vi "conditioning monitor.vi"() -> ()   [LabVIEW 2016, in "Top Level.lvlib"]
doc: "takes the teminal voltage as well as the vacuum values for both the entrance and exit of accelerator. Display\nboth in long terminal graph form. Every 24 hours, the graph is cleared."
uses:
  Top Level.lvlib
  Controls/Vertical Rod states.ctl
panel:
  out "Current Time":string
  in  "reset":bool
  out "error out 2":errorcluster
  out "Start Time":string
  out "error out":errorcluster
  out "Terminal Voltage":cluster{"X":dbl[], "Y":dbl[]}[](graph)
  out "Tank Vacuum Pressures":cluster{"X":dbl[], "Y":dbl[]}[](graph)
  in  "Cluster":cluster{"X":dbl[], "Y":dbl[]}
  in  "stop":bool
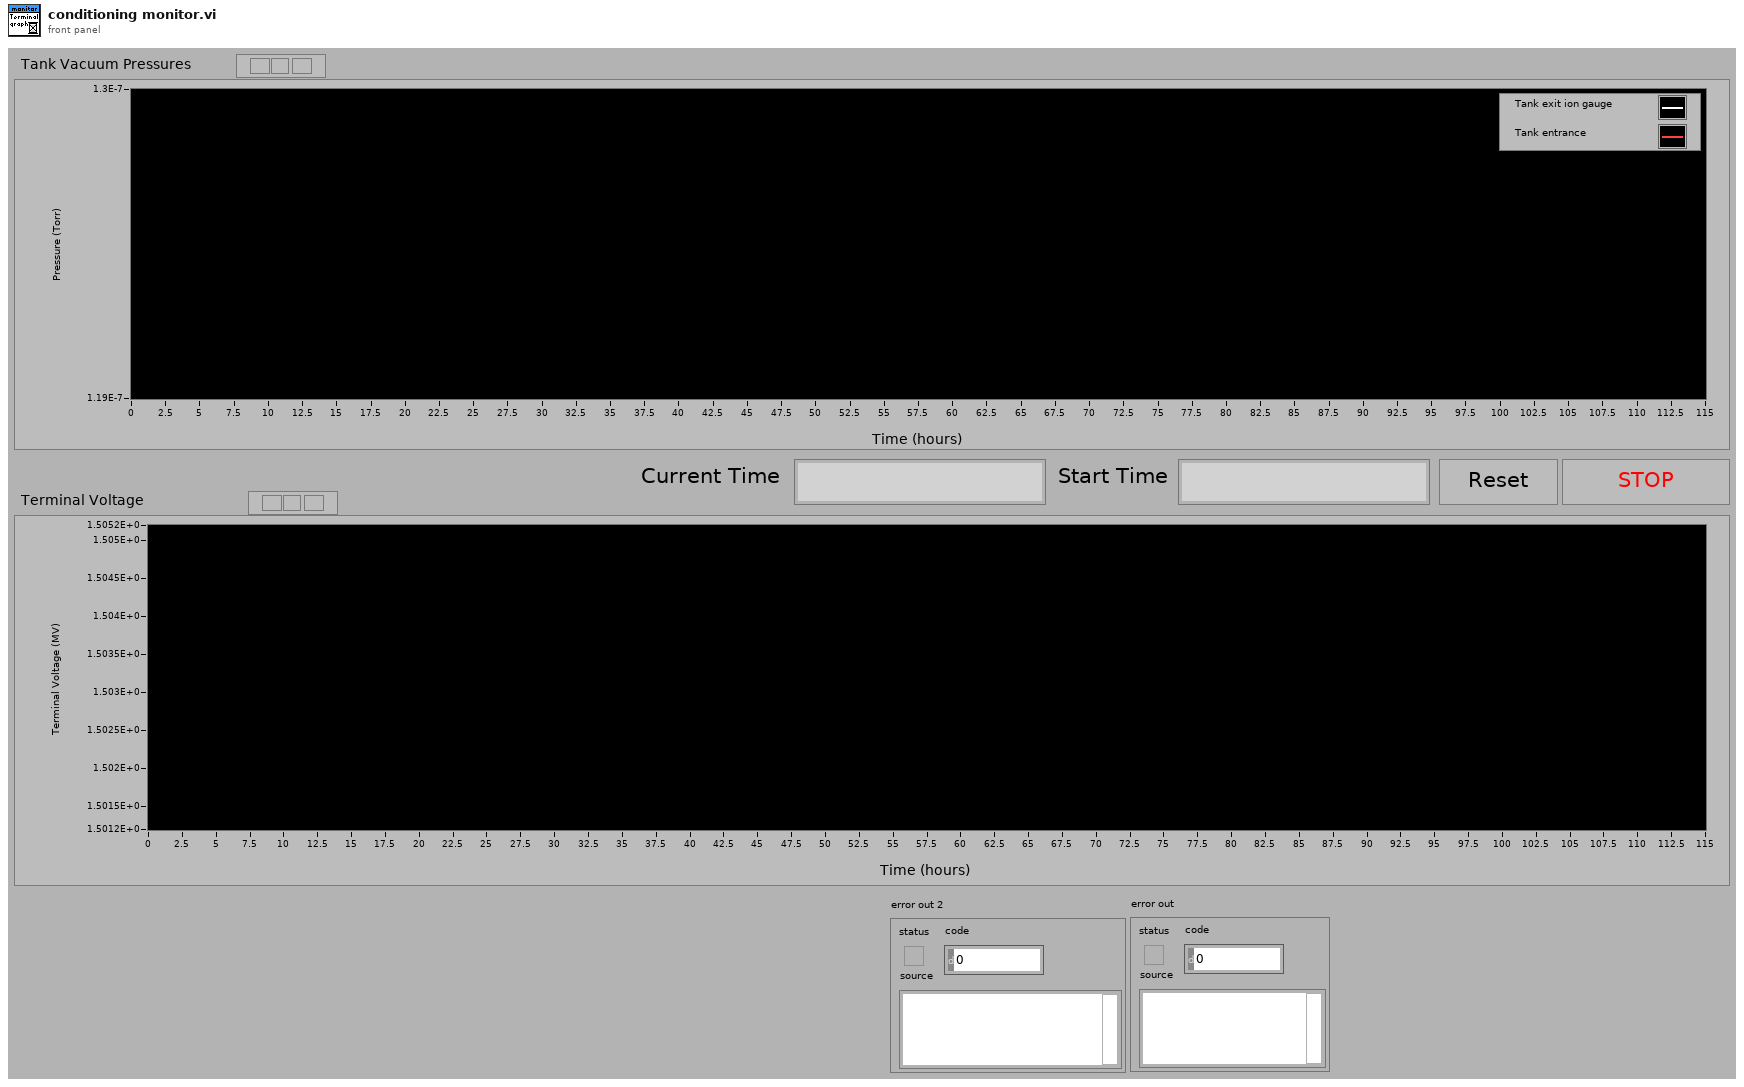
[diagram p1: front panel]
types:
  T1 = typedef "Vertical Rod states.ctl" = enum16{"status unclear", "rod down", "rod up"}
  T2 = cluster{"Ion gauge 1":string, "Convectron  Gauge 1 ":string, "Ion Gauge 2":string, "Convectrom Gauge 2":string}
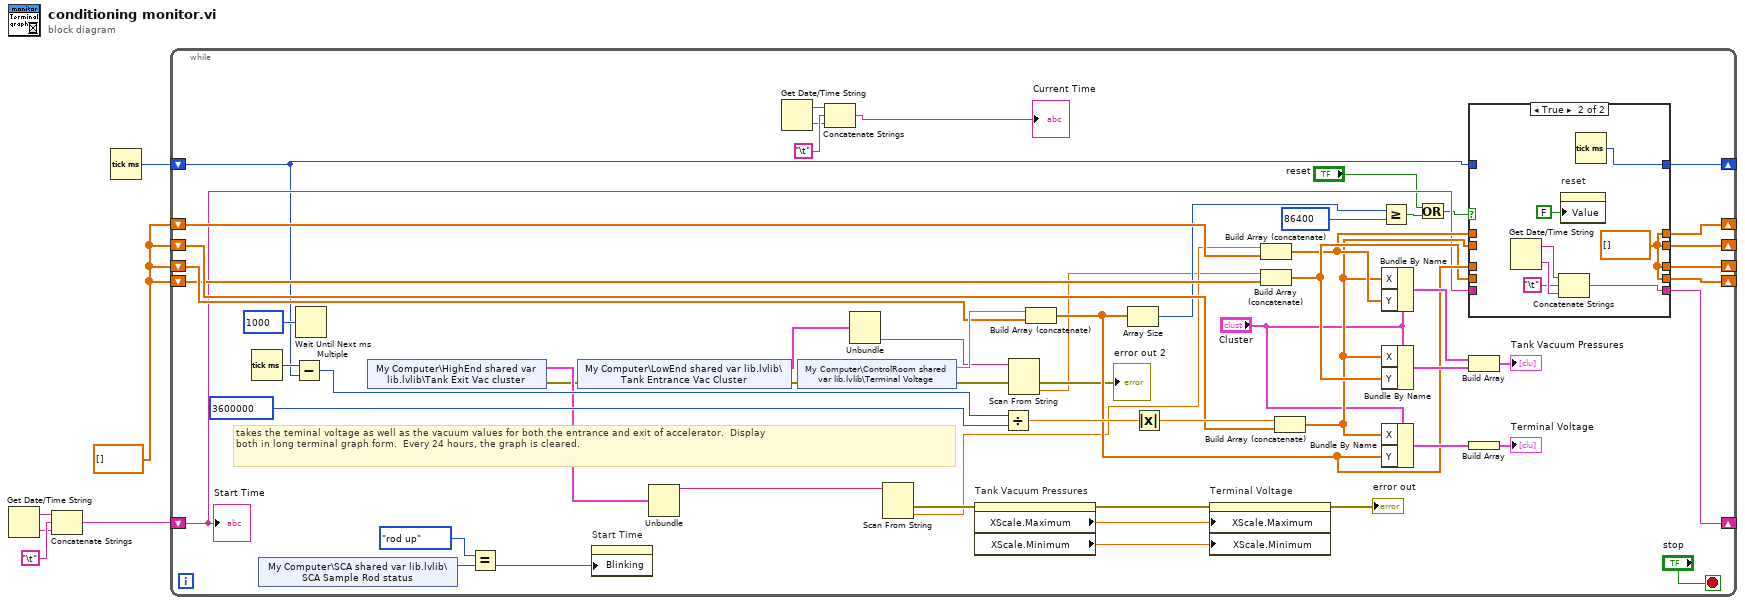
[diagram p0: block diagram]
diagram:
  w5 = dbl[] []
  n1 = Get Date/Time String() -> (date string=w4:string, time string=w2:string)  [unwired: 3 in]
  n2 = Concatenate Strings(w4, "\t", w2) -> (w1:string)
  n3 = Tick Count (ms)() -> (millisecond timer value=w6:u32)
  n4 = while {
    shift-right: [w27] -> _
    shift-left: w5 -> [w58]
    shift-right: [w25] -> _
    shift-left: w5 -> [w55]
    shift-right: [w31] -> _
    shift-left: w5 -> [w47]
    shift-right: [w29] -> _
    shift-left: w5 -> [w42]
    shift-right: [w24] -> _
    shift-left: w1 -> [w23]
    shift-right: [w13] -> _
    shift-left: w6 -> [w14]
    stop <- "stop" stop-if-true
    # "takes the teminal voltage as well as the vacuum values for both the entrance and exit of accelerator.  Display\nboth in long terminal graph form.  Every 24 hours, the graph is cleared."
    n5 = Tick Count (ms)() -> (millisecond timer value=w63:u32)
    n6 = shared-variable "My Computer\\SCA shared var lib.lvlib\\SCA Sample Rod status"() -> (w19:T1)  [unwired: 1 in, 1 out]
    n7 = Subtract(x=w63, y=w14) -> (x-y=w62:u32)
    n8 = Wait Until Next ms Multiple(millisecond multiple=u32 1000) -> ()  [unwired: 1 out]
    n9 = shared-variable "My Computer\\HighEnd shared var lib.lvlib\\Tank Exit Vac cluster"() -> (w52:T2, error out=w40:errorcluster)  [unwired: 1 in]
    n10 = Equal?(x=Vertical_Rod_states."rod up", y=w19) -> (x = y?=w8:bool)
    n11 = shared-variable "My Computer\\LowEnd shared var lib.lvlib\\Tank Entrance Vac Cluster"(error in=w40) -> (w44:T2, error out=w39:errorcluster)
    n12 = property on="Start Time" class="Str"("Blinking"=w8) -> ()  [unwired: 2 in, 2 out]
    n13 = Unbundle(w52) -> ("Ion gauge 1"=w51:string)  [unwired: 3 out]
    n14 = Get Date/Time String() -> (date string=w12:string, time string=w10:string)  [unwired: 3 in]
    n15 = shared-variable "My Computer\\ControlRoom shared var lib.lvlib\\Terminal Voltage"(error in=w39) -> (w49:dbl, error out=w38:errorcluster)
    n16 = Concatenate Strings(w12, "\t", w10) -> (→"Current Time":string)
    n17 = Unbundle(w44) -> ("Convectrom Gauge 2"=w43:string)  [unwired: 3 out]
    n18 = Scan From String(input string=w51) -> (error out=w37:errorcluster, output 1=w21:dbl)  [unwired: 4 in, 2 out]
    n19 = property on="Tank Vacuum Pressures" class="XYGraph (strict)"(error in=w37) -> (error out=w36:errorcluster, "XScale.Maximum"=w46:dbl, "XScale.Minimum"=w45:dbl)  [unwired: 1 in, 1 out]
    n20 = Divide(x=w62, y=u32 3600000) -> (x/y=w57:dbl)
    n21 = Scan From String(input string=w43, error in=w38) -> (error out=→"error out 2":errorcluster, output 1=w18:dbl)  [unwired: 3 in, 2 out]
    n22 = Build Array (concatenate)(w49, w47) -> (w32:dbl[])
    n23 = Array Size(array=w32) -> (size(s)=w34:i32)
    n24 = Absolute Value(x=w57) -> (abs(x)=w56:dbl)
    n25 = property on="Terminal Voltage" class="XYGraph (strict)"(error in=w36, "XScale.Maximum"=w46, "XScale.Minimum"=w45) -> (error out=→"error out":errorcluster)  [unwired: 1 in, 1 out]
    n26 = Build Array (concatenate)(w21, w58) -> (w28:dbl[])
    n27 = Build Array (concatenate)(w18, w42) -> (w30:dbl[])
    n28 = Build Array (concatenate)(w56, w55) -> (w26:dbl[])
    n29 = Greater Or Equal?(x=w34, y=86400) -> (x >= y?=w16:bool)
    n30 = Bundle By Name(cluster="Cluster", "X"=w26, "Y"=w28) -> (w54:cluster{"X":dbl[], "Y":dbl[]})
    n31 = Bundle By Name(cluster="Cluster", "X"=w26, "Y"=w30) -> (w41:cluster{"X":dbl[], "Y":dbl[]})
    n32 = Bundle By Name(cluster="Cluster", "X"=w26, "Y"=w32) -> (w50:cluster{"X":dbl[], "Y":dbl[]})
    n33 = Or(x="reset", y=w16) -> (x .or. y?=w17:bool)
    n34 = case shown="True" w17 {
      tunnel: w32 -> [w69 _]
      tunnel: [w69 w76] -> w31
      tunnel: w30 -> [w68 _]
      tunnel: [w68 w76] -> w29
      tunnel: w28 -> [w67 _]
      tunnel: [w67 w76] -> w27
      tunnel: w26 -> [w66 _]
      tunnel: [w66 w76] -> w25
      tunnel: [w65 w72] -> w24
      tunnel: w23 -> [w65 _]
      tunnel: w14 -> [w64 _]
      tunnel: [w64 w70] -> w13
      frame False {
      }
      frame True {
        w76 = dbl[] []
        n35 = Get Date/Time String() -> (date string=w73:string, time string=w75:string)  [unwired: 3 in]
        n36 = Concatenate Strings(w73, "\t", w75) -> (w72:string)
        n37 = property on="reset" class="Bool (strict)"("Value"=FALSE ("reset")) -> ()  [unwired: 2 in, 2 out]
        n38 = Tick Count (ms)() -> (millisecond timer value=w70:u32)
      }
    }
    n39 = Build Array(w54, w41) -> (→"Tank Vacuum Pressures":cluster{"X":dbl[], "Y":dbl[]}[])
    n40 = Build Array(w50) -> (→"Terminal Voltage":cluster{"X":dbl[], "Y":dbl[]}[])
    "Start Time" <- w23
  }
